vi "Write Display String Event.vi"(8 "error in (no error)":errorcluster, 10 "Display String Event":T1, 11 "Stock Trader in":refnum<class "Stock Trader.lvclass">) -> (0 "error out":errorcluster, 3 "Stock Trader out":refnum<class "Stock Trader.lvclass">)   [LabVIEW 2019, in "Stock Trader.lvclass"]
doc: "Set Display String Event. The Display string user event accepts a string and when received updates the front panel's display string."
uses:
  Stock Trader.lvclass
  Controls/Display Event.ctl
  Stock Trader.lvclass/Stock Trader.ctl
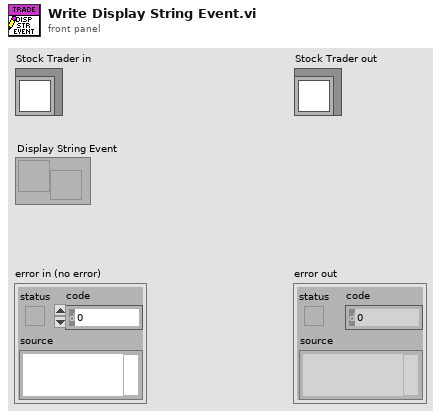
[diagram p1: front panel]
types:
  T1 = typedef "Display Event.ctl" = refnum<user-event>
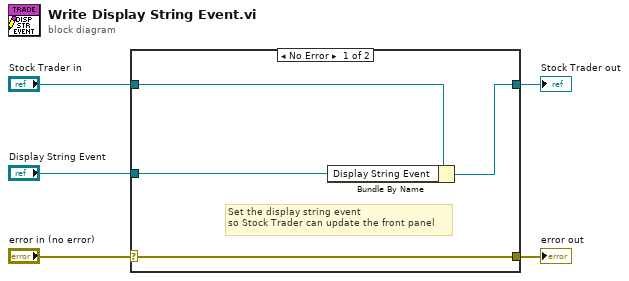
[diagram p0: block diagram]
diagram:
  n1 = case shown="No Error" "error in (no error)" {
    selector: "error in (no error)" -> [w9 w10]
    tunnel: [w9 w10] -> w4
    tunnel: [w7 w11] -> w2
    tunnel: "Stock Trader in" -> [w8 w11]
    tunnel: "Display String Event" -> [w6 _]
    frame No Error {
      # "Set the display string event \nso Stock Trader can update the front panel"
      n2 = Bundle By Name(cluster=w8, "Display String Event"=w6) -> (w7:refnum<class "Stock Trader.lvclass">)
    }
    frame Error {
    }
  }
  "error out" <- w4
  "Stock Trader out" <- w2
